vi "TEST - Format Variant Into String.vi"(8 "error in (no error)":errorcluster) -> (0 "error out":errorcluster, 2 "Pass":bool)   [LabVIEW 2009]
panel:
  out "Failures":T1(array[cluster])
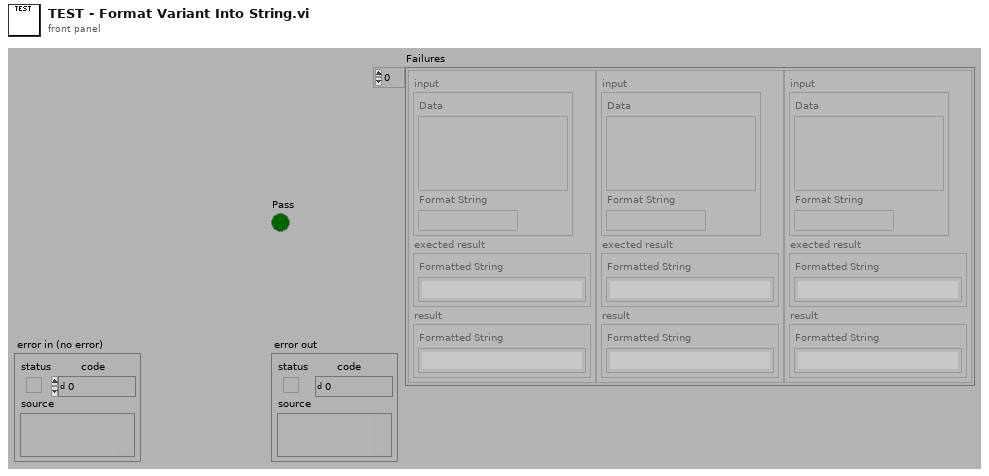
[diagram p1: front panel]
types:
  T1 = cluster{"input":cluster{"Data":variant, "Format String":string}, "exected result":cluster{"Formatted String":string}, "result":cluster{"Formatted String":string}}[]
  T2 = cluster{"input":cluster{"Data":variant, "Format String":string}, "exected result":cluster{"Formatted String":string}, "result":cluster{"Formatted String":string}}
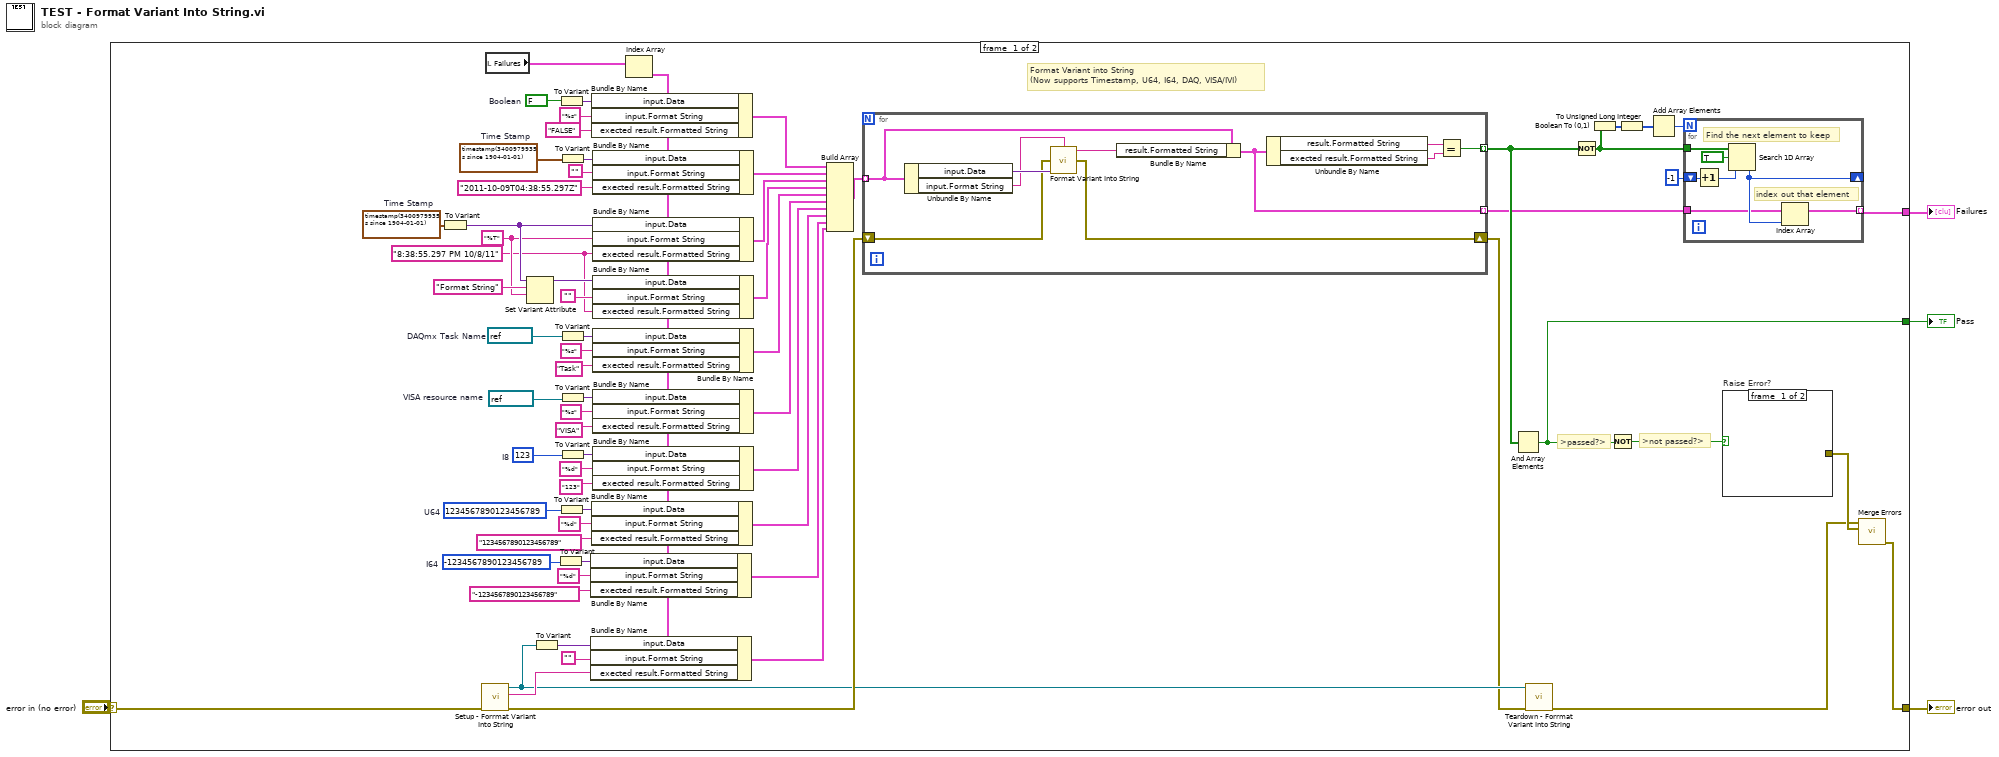
[diagram p0: block diagram]
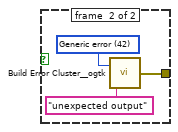
[diagram p2: hidden frame]
diagram:
  n1 = case shown="No Error" "error in (no error)" {
    selector: "error in (no error)" -> [w10 w93]
    tunnel: [w48 _] -> w4
    tunnel: [w72 w93] -> w2
    tunnel: [w63 _] -> w1
    frame #0 {
      w15 = "8:38:55.297 PM 10/8/11" ("y")
      w19 = "%T" ("format string")
      w26 = timestamp(3400979935.297 s since 1904-01-01)  # Time Stamp
      w28 = i64 -1234567890123456789  # I64
      w38 = u64 1234567890123456789  # U64
      w39 = i8 123  # I8
      w42 = refnum<visa-resource-name> "VISA"  # VISA resource name
      w50 = refnum<k21> "Task"  # DAQmx Task Name
      w69 = FALSE  # Boolean
      w56 = timestamp(3400979935.297 s since 1904-01-01)  # Time Stamp
      # "Format Variant into String\n(Now supports Timestamp, U64, I64, DAQ, VISA/IVI)"
      # ">not passed?>"
      # ">passed?>"
      n2 = To Variant(anything=w26) -> (Variant=w21:variant)
      n3 = call "Setup - Forrmat Variant Into String.vi"("error in (no error)"=w10) -> ("error out"=w9:errorcluster, "Input String"=w8:string, "Refnum"=w7:refnum<file>)  [unwired: 8 in]
      n4 = local read "Failures"() -> (w62:T1)
      n5 = Set Variant Attribute(Variant=w21, name="Format String", value=w19) -> (Variant out=w18:variant)  [unwired: 1 in, 2 out]
      n6 = To Variant(anything=w7) -> (Variant=w14:variant)
      n7 = To Variant(anything=w28) -> (Variant=w31:variant)
      n8 = To Variant(anything=w69) -> (Variant=w61:variant)
      n9 = To Variant(anything=w38) -> (Variant=w35:variant)
      n10 = To Variant(anything=w56) -> (Variant=w57:variant)
      n11 = To Variant(anything=w50) -> (Variant=w54:variant)
      n12 = To Variant(anything=w42) -> (Variant=w44:variant)
      n13 = To Variant(anything=w39) -> (Variant=w41:variant)
      n14 = Index Array(array=w62) -> (element=w12:T2)  [unwired: 1 in]
      n15 = Bundle By Name(cluster=w12, "input.Data"=w31, "input.Format String"="%d" ("format string"), "exected result.Formatted String"="-1234567890123456789" ("y")) -> (w27:T2)
      n16 = Bundle By Name(cluster=w12, "input.Data"=w14, "input.Format String"="", "exected result.Formatted String"=w8) -> (w13:T2)
      n17 = Bundle By Name(cluster=w12, "input.Data"=w61, "input.Format String"="%s" ("format string"), "exected result.Formatted String"="FALSE" ("y")) -> (w55:T2)
      n18 = Bundle By Name(cluster=w12, "input.Data"=w35, "input.Format String"="%d" ("format string"), "exected result.Formatted String"="1234567890123456789" ("y")) -> (w32:T2)
      n19 = Bundle By Name(cluster=w12, "input.Data"=w57, "input.Format String"="", "exected result.Formatted String"="2011-10-09T04:38:55.297Z" ("y")) -> (w25:T2)
      n20 = Bundle By Name(cluster=w12, "input.Data"=w21, "input.Format String"=w19, "exected result.Formatted String"=w15) -> (w24:T2)
      n21 = Bundle By Name(cluster=w12, "input.Data"=w18, "input.Format String"="", "exected result.Formatted String"=w15) -> (w22:T2)
      n22 = Bundle By Name(cluster=w12, "input.Data"=w54, "input.Format String"="%s" ("format string"), "exected result.Formatted String"="Task" ("y")) -> (w23:T2)
      n23 = Bundle By Name(cluster=w12, "input.Data"=w44, "input.Format String"="%s" ("format string"), "exected result.Formatted String"="VISA" ("y")) -> (w43:T2)
      n24 = Bundle By Name(cluster=w12, "input.Data"=w41, "input.Format String"="%d" ("format string"), "exected result.Formatted String"="123" ("y")) -> (w33:T2)
      n25 = Build Array(w55, w25, w24, w22, w23, w43, w33, w32, w27, w13) -> (w51:T1)
      n26 = for {
        tunnel: w51 -> [w86] mode=indexing
        shift-right: [w88] -> w6
        shift-left: w9 -> [w87]
        tunnel: [w83] -> w49 mode=indexing
        tunnel: [w80] -> w47 mode=indexing
        n27 = Unbundle By Name(w86) -> ("input.Data"=w89:variant, "input.Format String"=w84:string)
        n28 = call "Format Variant Into String.vi"("Format String"=w84, "error in (no error)"=w87, "Variant"=w89) -> ("Output String"=w85:string, "error out"=w88:errorcluster)  [unwired: 11 in]
        n29 = Bundle By Name(cluster=w86, "result.Formatted String"=w85) -> (w80:T2)
        n30 = Unbundle By Name(w80) -> ("result.Formatted String"=w82:string, "exected result.Formatted String"=w81:string)
        n31 = Equal?(x=w82, y=w81) -> (x = y?=w83:bool)
      }
      n32 = And Array Elements(Boolean array=w49) -> (logical AND=w48:bool)
      n33 = call "Teardown - Forrmat Variant Into String.vi"("error in (no error)"=w6, "Refnum"=w7) -> ("error out"=w5:errorcluster)  [unwired: 9 in]
      n34 = Not(x=w49) -> (.not. x?=w65:bool[])
      n35 = Boolean To (0,1)(Boolean=w65) -> (0, 1=w66:i16[])
      n36 = Not(x=w48) -> (.not. x?=w70:bool)
      n37 = To Unsigned Long Integer(number=w66) -> (unsigned 32bit integer=w64:u32[])
      n38 = Add Array Elements(numeric array=w64) -> (sum=w67:u32)
      n39 = for {
        N: w67 -> [_]
        tunnel: w47 -> [w75]
        tunnel: w65 -> [w79]
        shift-right: [w76] -> _
        shift-left: -1 ("start index (0)") -> [w77]
        tunnel: [w74] -> w63 mode=indexing
        # "index out that element"
        # "Find the next element to keep"
        n40 = Increment(x=w77) -> (x+1=w73:i32)
        n41 = Search 1D Array(1D array=w79, element=TRUE, start index (0)=w73) -> (index of element=w76:i32)
        n42 = Index Array(array=w75, index=w76) -> (element=w74:T2)
      }
      n43 = case "Raise Error?" shown="True" w70 {
        tunnel: [_ w90] -> w71
        frame #0 {
        }
        frame #1 {
          w91 = 42 items=["No error", "Argument error", "Memory is full", "Out of zone", "End of file", "File already open", "Generic file I/O error", "File not found", "File permission error", "Disk is full", "Duplicate path", "Too many files open", "System feature not enabled", "Resource file not found", "Cannot add resource", "Resource not found", "Image not found", "Image memory error", "Pen does not exist", "Config type invalid", "Config token not found", "Config parse error", "Config memory error", "Bad external code format", "Bad external code offset", "External code not present", "Null window", "Destroy window error", "Null menu", "Print aborted", "Bad print record", "Print driver error", "Windows error during printing", "Memory error during printing", "Print dialog error", "Generic print error", "Invalid device refnum", "Device not found", "Device parameter error", "Device unit error", "Cannot open device", "Device call aborted", "Generic error", "Cancelled by user", "Object ID too low", "Object ID too high", "Object not in heap", "Unknown heap", "Unknown object (invalid DefProc)", "Unknown object (DefProc not in table)", "Message out of range", "Invalid (null) method", "Unknown message", "Manager call not supported", "Bad address", "Network operation in progress", "Network operation timed out", "Connection is busy", "Network attribute not supported", "Network error", "Address in use", "System out of memory", "Connection aborted", "Connection refused", "Not connected", "Already connected", "Connection closed", "Initialization error (interapplication manager)", "Bad occurrence", "Wait on unbound occurrence handler", "Occurrence queue overflow", "Datalog type conflict", "Unused", "Unrecognized type (interapplication manager)", "Memory corrupt", "Failed to make temporary DLL", "Old CIN version", "Drag socket not found", "Failed to load drop-object", "Failed to register OLE object", "Failed to release OLE object", "Format specifier type mismatch", "Unknown format specifier", "Too few format specifiers", "Too many format specifiers", "Scan failed", "Newer CIN version", "Error converting to variant", "Runtime menu error", "Password tampered", "Variant attribute not found", "Incompatible variant data type", "Event data is not available", "Event Store is not present", "Occurrence is not found", "Event Queue is not created", "Event info is not available", "Refnum passed is NULL", "Error retrieving Class GUID", "Error retrieving CoClass GUID", "Error retrieving TypeLib GUID.", "Bad built application magic bytes.", "Specific driver is different from the specific driver associated with the Logical Name.", "There is no session opened to the class driver.", "Max Error", "MAX - Error with config objects", "MAX - Error loading configuration", "MAX - Group not supported"]
          n44 = call <userlib>:"Build Error Cluster__ogtk.vi"("String to Prepend to source (\"\")"="unexpected output" ("String to Prepend to source (\"\")"), "code"=w91) -> ("error out"=w90:errorcluster)
        }
      }
      n45 = call <vilib>:"Merge Errors.vi"("error in 2 (no error)"=w71, "error in 1 (no error)"=w5) -> ("error out"=w72:errorcluster)  [unwired: 5 in]
    }
    frame #1 {
    }
  }
  "Pass" <- w4
  "error out" <- w2
  "Failures" <- w1
